vi "Pre Launch Init.vi"(11 "DataLogger in":refnum<class "DataLogger.lvclass">) -> (0 "error out":errorcluster, 3 "DataLogger out":refnum<class "DataLogger.lvclass">)   [LabVIEW 2019, in "DataLogger.lvclass"]
doc: "(<B>Filename</B>: Actor Framework.lvlib:Actor.lvclass:Pre Launch Init.vi)\n\nDefines behavior that occurs after the Launch Nested Actor method is invoked but before the actor's Actor Core method begins running.\n\nBy default, this method does nothing. A descendant class may override it to define behavior."
uses:
  DataLogger.lvclass
  <vilib>/ActorFramework/Actor/Actor.lvclass
  <vilib>/vision/Image Controls.llb/IMAQ Image.ctl
  Common/Controls/AllPartInfo.ctl
panel:
  in  "MasterSampleInfo":T1
  in  "LogMeasurementData":bool
  in  "BatchID":string
  in  "MachineStatus":string
  in  "Measurement Info":T2
  in  "PartDetails":T3
  in  "AllPartInfoArray":T4=[{"PartName"="", "NumberOfRacks"=0, "MeasurementIDsArray"=[], "MeasurementNamesArray"=[], "SpecValuesArray"=[]}]
  in  "Statistical Info":T5
  in  "State Message":string
  in  "Batch Info":T6
  in  "Failure Info":T8
  in  "Event Info":T9
  in  "Reel Info":T10
  in  "Part Info":T11
  in  "System Info":T12
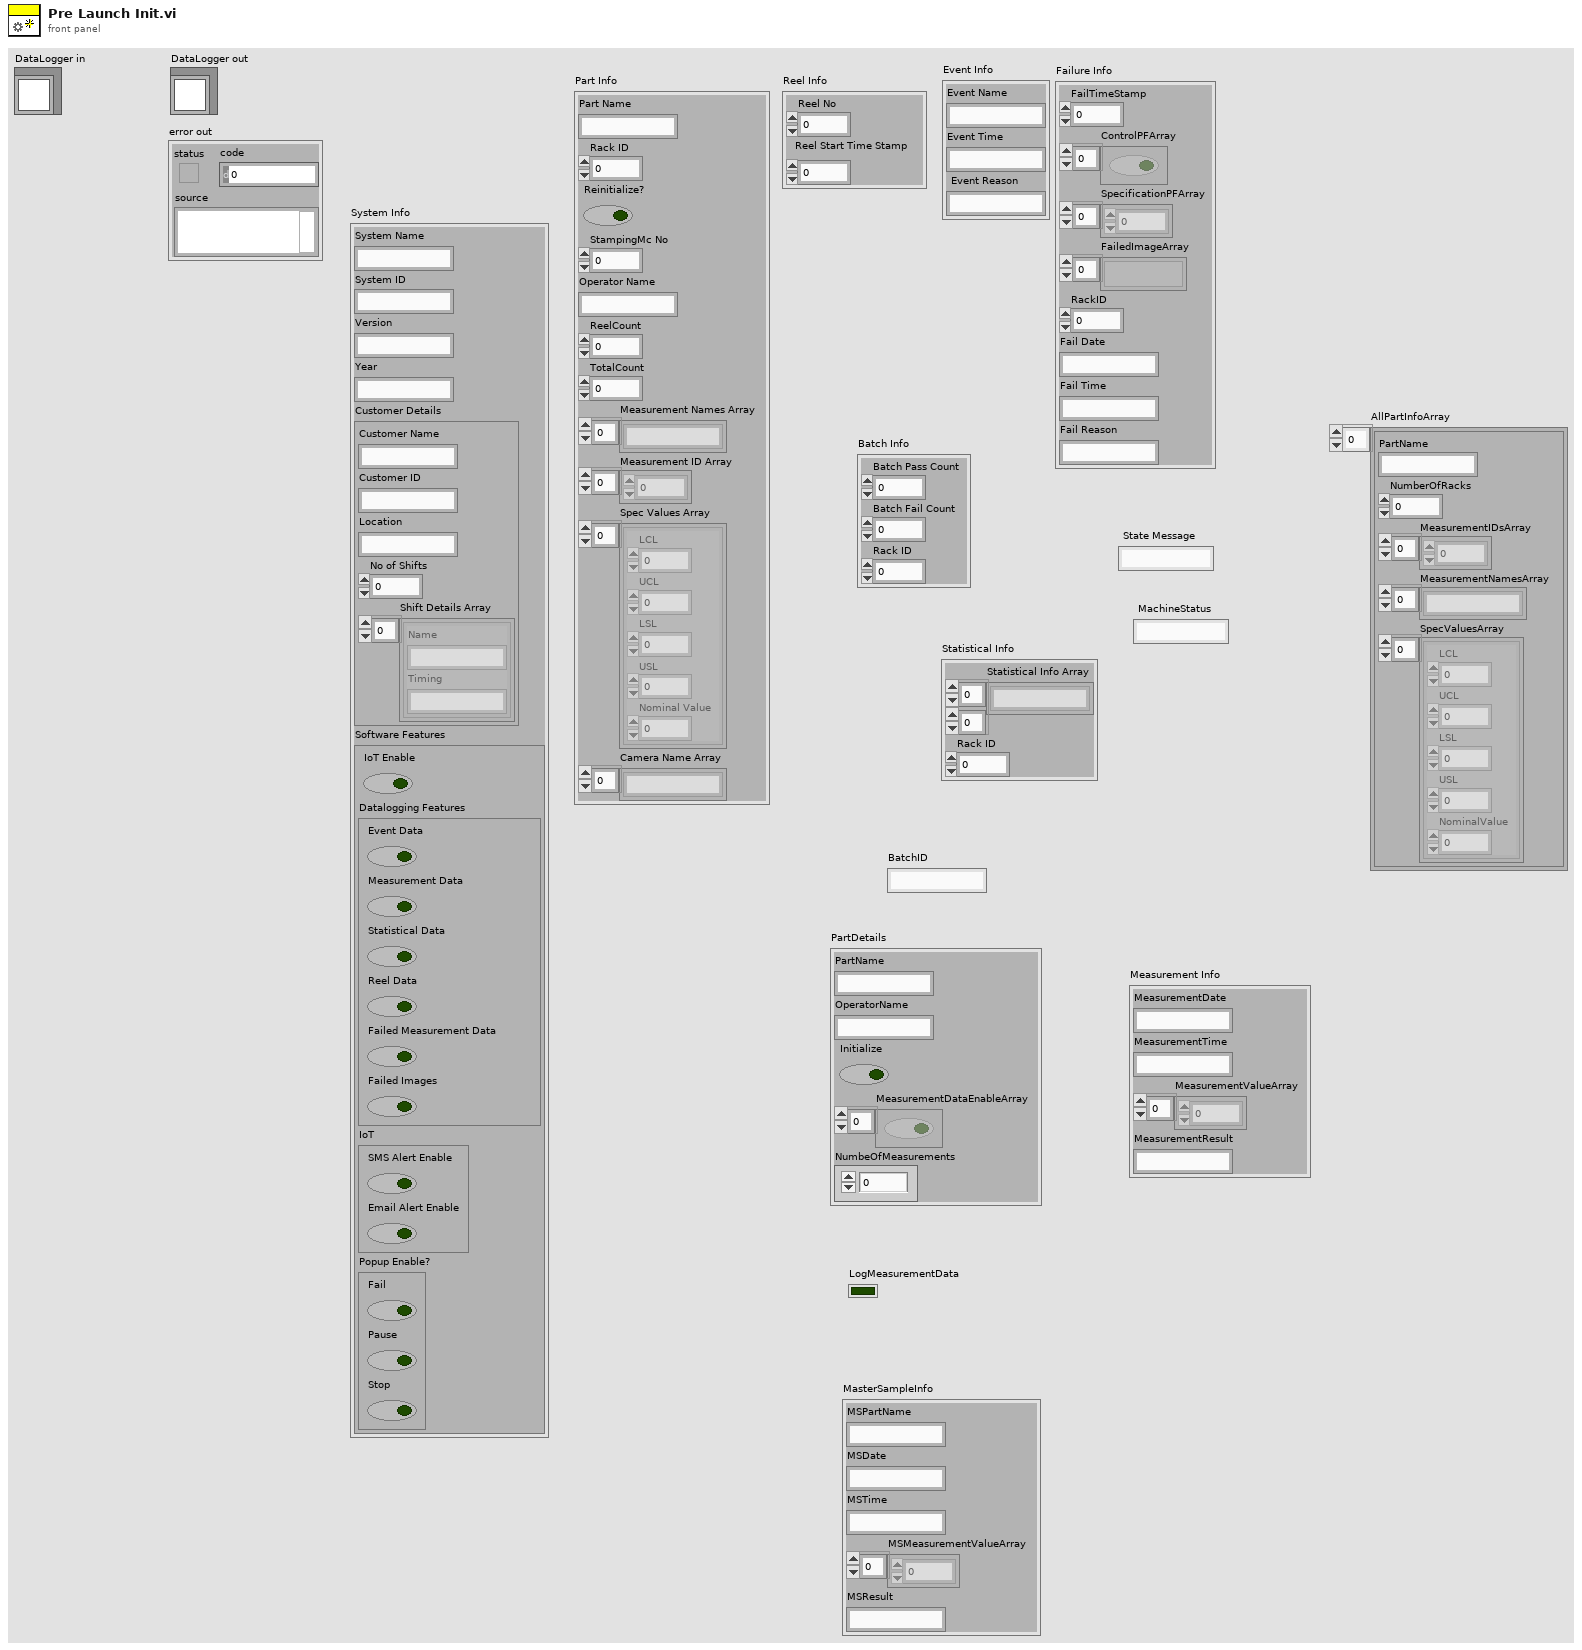
[diagram p1: front panel]
types:
  T1 = cluster{"MSPartName":string, "MSDate":string, "MSTime":string, "MSMeasurementValueArray":dbl[], "MSResult":string}
  T2 = cluster{"MeasurementDate":string, "MeasurementTime":string, "MeasurementValueArray":dbl[], "MeasurementResult":string}
  T3 = cluster{"PartName":string, "OperatorName":string, "Initialize":bool, "MeasurementDataEnableArray":bool[], "NumbeOfMeasurements":i32}
  T4 = typedef "AllPartInfo.ctl" = cluster{"PartName":string, "NumberOfRacks":u8, "MeasurementIDsArray":u16[], "MeasurementNamesArray":string[], "SpecValuesArray":cluster{"LCL":dbl, "UCL":dbl, "LSL":dbl, "USL":dbl, "NominalValue":dbl}[]}[]
  T5 = cluster{"Statistical Info Array":string[][], "Rack ID":u8}
  T6 = cluster{"Batch Pass Count":u64, "Batch Fail Count":u64, "Rack ID":u8}
  T7 = typedef "IMAQ Image.ctl" = refnum<image>
  T8 = cluster{"FailTimeStamp":u64, "ControlPFArray":bool[], "SpecificationPFArray":dbl[], "FailedImageArray":T7[], "RackID":u8, "Fail Date":string, "Fail Time":string, "Fail Reason":string}
  T9 = cluster{"Event Name":string, "Event Time":string, "Event Reason":string}
  T10 = cluster{"Reel No":u64, "Reel Start Time Stamp":u64}
  T11 = cluster{"Part Name":string, "Rack ID":u8, "Reinitialize?":bool, "StampingMc No":u64, "Operator Name":string, "ReelCount":u64, "TotalCount":u64, "Measurement Names Array":string[], "Measurement ID Array":u16[], "Spec Values Array":cluster{"LCL":dbl, "UCL":dbl, "LSL":dbl, "USL":dbl, "Nominal Value":dbl}[], "Camera Name Array":string[]}
  T12 = cluster{"System Name":string, "System ID":string, "Version":string, "Year":string, "Customer Details":cluster{"Customer Name":string, "Customer ID":string, "Location":string, "No of Shifts":u8, "Shift Details Array":cluster{"Name":string, "Timing":string}[]}, "Software Features":cluster{"IoT Enable":bool, "Datalogging Features":cluster{"Event Data":bool, "Measurement Data":bool, "Statistical Data":bool, "Reel Data":bool, "Failed Measurement Data":bool, "Failed Images":bool}, "IoT":cluster{"SMS Alert Enable":bool, "Email Alert Enable":bool}, "Popup Enable?":cluster{"Fail":bool, "Pause":bool, "Stop":bool}}}
  T13 = cluster{"Shift Name":string, "Shift Timing":string, "Shift End Date":string, "Statistical Shift Data":cluster{"PartName":string, "MeasurementNames":string[], "Statistical Parameters":string[][]}[]}
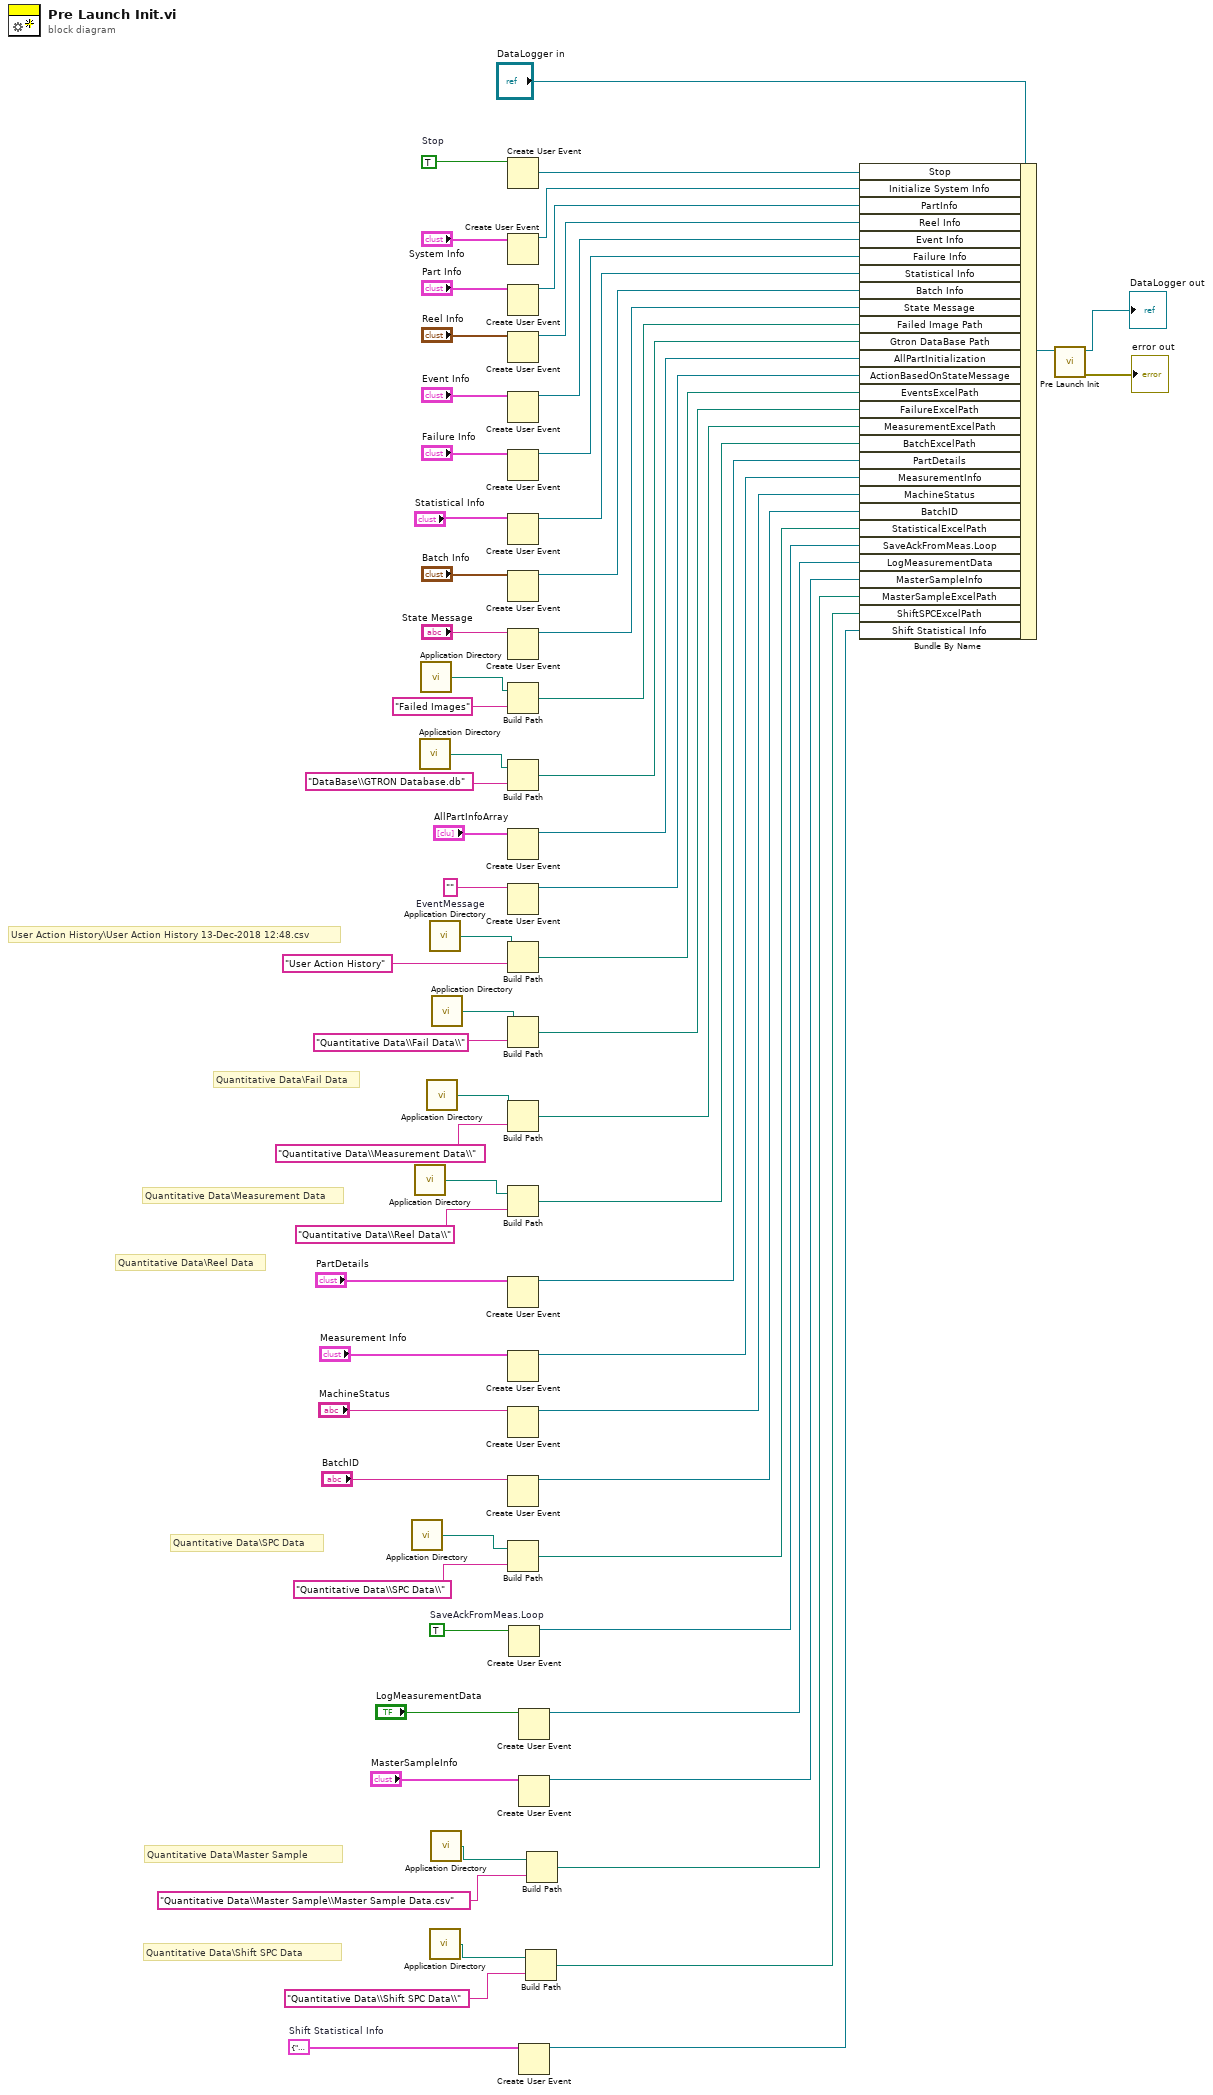
[diagram p0: block diagram]
diagram:
  w2 = T13 {"Shift Name"="", "Shift Timing"="", "Shift End Date"="", "Statistical Shift Data"=[]}  # Shift Statistical Info
  w16 = TRUE  # SaveAckFromMeas.Loop
  w44 = ""  # EventMessage
  w67 = TRUE  # Stop
  # "Quantitative Data\\Shift SPC Data"
  # "Quantitative Data\\Master Sample"
  # "User Action History\\User Action History 13-Dec-2018 12:48.csv"
  # "Quantitative Data\\SPC Data"
  # "Quantitative Data\\Reel Data"
  # "Quantitative Data\\Fail Data"
  # "Quantitative Data\\Measurement Data"
  n1 = call <vilib>:"Application Directory.vi"() -> ("Application Directory"=w19:path)
  n2 = call <vilib>:"Application Directory.vi"() -> ("Application Directory"=w36:path)
  n3 = call <vilib>:"Application Directory.vi"() -> ("Application Directory"=w47:path)
  n4 = call <vilib>:"Application Directory.vi"() -> ("Application Directory"=w51:path)
  n5 = call <vilib>:"Application Directory.vi"() -> ("Application Directory"=w39:path)
  n6 = call <vilib>:"Application Directory.vi"() -> ("Application Directory"=w42:path)
  n7 = call <vilib>:"Application Directory.vi"() -> ("Application Directory"=w4:path)
  n8 = call <vilib>:"Application Directory.vi"() -> ("Application Directory"=w8:path)
  n9 = call <vilib>:"Application Directory.vi"() -> ("Application Directory"=w40:path)
  n10 = Create User Event(user event datatype=w67) -> (user event=w65:refnum<user-event>)  [unwired: 1 in, 1 out]
  n11 = Create User Event(user event datatype="System Info") -> (user event=w27:refnum<user-event>)  [unwired: 1 in, 1 out]
  n12 = Create User Event(user event datatype="Part Info") -> (user event=w30:refnum<user-event>)  [unwired: 1 in, 1 out]
  n13 = Create User Event(user event datatype="Reel Info") -> (user event=w29:refnum<user-event>)  [unwired: 1 in, 1 out]
  n14 = Create User Event(user event datatype="Event Info") -> (user event=w59:refnum<user-event>)  [unwired: 1 in, 1 out]
  n15 = Create User Event(user event datatype="Failure Info") -> (user event=w28:refnum<user-event>)  [unwired: 1 in, 1 out]
  n16 = Create User Event(user event datatype="Statistical Info") -> (user event=w53:refnum<user-event>)  [unwired: 1 in, 1 out]
  n17 = Create User Event(user event datatype="Batch Info") -> (user event=w52:refnum<user-event>)  [unwired: 1 in, 1 out]
  n18 = Create User Event(user event datatype="State Message") -> (user event=w55:refnum<user-event>)  [unwired: 1 in, 1 out]
  n19 = Build Path(base path=w51, name or relative path="Failed Images") -> (appended path=w49:path)
  n20 = Build Path(base path=w47, name or relative path="DataBase\\GTRON Database.db") -> (appended path=w46:path)
  n21 = Create User Event(user event datatype="AllPartInfoArray") -> (user event=w31:refnum<user-event>)  [unwired: 1 in, 1 out]
  n22 = Create User Event(user event datatype=w44) -> (user event=w43:refnum<user-event>)  [unwired: 1 in, 1 out]
  n23 = Build Path(base path=w42, name or relative path="User Action History") -> (appended path=w35:path)
  n24 = Build Path(base path=w40, name or relative path="Quantitative Data\\Fail Data\\") -> (appended path=w34:path)
  n25 = Build Path(base path=w39, name or relative path="Quantitative Data\\Measurement Data\\") -> (appended path=w33:path)
  n26 = Build Path(base path=w36, name or relative path="Quantitative Data\\Reel Data\\") -> (appended path=w32:path)
  n27 = Create User Event(user event datatype="PartDetails") -> (user event=w11:refnum<user-event>)  [unwired: 1 in, 1 out]
  n28 = Create User Event(user event datatype="Measurement Info") -> (user event=w24:refnum<user-event>)  [unwired: 1 in, 1 out]
  n29 = Create User Event(user event datatype="MachineStatus") -> (user event=w22:refnum<user-event>)  [unwired: 1 in, 1 out]
  n30 = Create User Event(user event datatype="BatchID") -> (user event=w20:refnum<user-event>)  [unwired: 1 in, 1 out]
  n31 = Build Path(base path=w19, name or relative path="Quantitative Data\\SPC Data\\") -> (appended path=w17:path)
  n32 = Create User Event(user event datatype=w16) -> (user event=w14:refnum<user-event>)  [unwired: 1 in, 1 out]
  n33 = Create User Event(user event datatype="LogMeasurementData") -> (user event=w12:refnum<user-event>)  [unwired: 1 in, 1 out]
  n34 = Create User Event(user event datatype="MasterSampleInfo") -> (user event=w9:refnum<user-event>)  [unwired: 1 in, 1 out]
  n35 = Create User Event(user event datatype=w2) -> (user event=w1:refnum<user-event>)  [unwired: 1 in, 1 out]
  n36 = Build Path(base path=w4, name or relative path="Quantitative Data\\Shift SPC Data\\") -> (appended path=w3:path)
  n37 = Build Path(base path=w8, name or relative path="Quantitative Data\\Master Sample\\Master Sample Data.csv") -> (appended path=w6:path)
  n38 = Bundle By Name(cluster="DataLogger in", "Stop"=w65, "Initialize System Info"=w27, "PartInfo"=w30, "Reel Info"=w29, "Event Info"=w59, "Failure Info"=w28, "Statistical Info"=w53, "Batch Info"=w52, "State Message"=w55, "Failed Image Path"=w49, "Gtron DataBase Path"=w46, "AllPartInitialization"=w31, "ActionBasedOnStateMessage"=w43, "EventsExcelPath"=w35, "FailureExcelPath"=w34, "MeasurementExcelPath"=w33, "BatchExcelPath"=w32, "PartDetails"=w11, "MeasurementInfo"=w24, "MachineStatus"=w22, "BatchID"=w20, "StatisticalExcelPath"=w17, "SaveAckFromMeas.Loop"=w14, "LogMeasurementData"=w12, "MasterSampleInfo"=w9, "MasterSampleExcelPath"=w6, "ShiftSPCExcelPath"=w3, "Shift Statistical Info"=w1) -> (w63:refnum<class "DataLogger.lvclass">)
  n39 = call-parent "Pre Launch Init.vi"("Actor in"=w63) -> ("error out"=→"error out":errorcluster, "Actor out"=→"DataLogger out":refnum<class "DataLogger.lvclass">)  [unwired: 9 in]
